vi "HOST_timecycling+4inputs.vi"() -> ()   [LabVIEW 2020]
uses:
  <vilib>/userDefined/Silver/nirio_resource_slv.ctl
  Controls/Clock Select.ctl
  <vilib>/FPGAPlugInAG/PXIe-7972R/niLvFpga_Open_PXIe-7972R.vi
  <vilib>/rvi/interface/common/dynamic/niFpgaDynamicAddResources.vi
  <vilib>/rvi/interface/common/niFpgaWaitOnOcc.vi
  <vilib>/Utility/error.llb/Error Cluster From Error Code.vi
  <vilib>/rvi/errors/niLvFpgaAdjustHostInterfaceError.vi
  <instrlib>/_niInstr/Streaming/v1/Host/Public/Start Finite Stream.vi
  <instrlib>/_niInstr/Streaming/v1/Host/Public/Wait for Stream.vi
  <instrlib>/_niInstr/Streaming/v1/Host/Public/Start Continuous Stream.vi
  <vilib>/FPGAPlugInAG/Dynamic/niLvFpga_Close_Dynamic.vi
  <vilib>/rvi/interface/nirviOpenFPGA/nirviOpenFPGA.xnode
  FPGA Bitfiles/rfsignal_FPGATarget_timecycling+4inp_VE6nLnBZ2oA.lvbitx
  <vilib>/rvi/interface/nirviMethod/nirviMethod.xnode
  <vilib>/rvi/interface/nirviReadWriteControl/nirviReadWriteControl.xnode
  <vilib>/rvi/interface/nirviCloseFPGA/nirviCloseFPGA.xnode
  <vilib>/rvi/errors/niLvFpgaMergeErrorWithErrorCode.vi
  <instrlib>/_niInstr/Streaming/v1/Host/niInstr Streaming v1 Host.lvlib
  <vilib>/rvi/interface/Simulation/niFpgaSimulationCallBeginRW.vi
  NiFpgaLv.dll
  <vilib>/FPGAPlugInAG/Dynamic/niLvFpga_ConfigureFifo_Dynamic.vi
  <vilib>/FPGAPlugInAG/Dynamic/niLvFpga_StartFifo_Dynamic.vi
  <vilib>/FPGAPlugInAG/Dynamic/niLvFpga_WriteFifo_Dynamic.vi
panel:
  in  "Feedback on/off":bool=TRUE
  in  "Scaling (Z)":fxp<+,5,-13>=9.918212890625e-05
  in  "Scaling (Y)":fxp<+,5,-13>=9.918212890625e-05
  in  "Scaling (X)":fxp<+,5,-13>=9.918212890625e-05
  in  "D (Z)":fxp<+/-,16,16>
  in  "I (Z)":fxp<+/-,16,16>
  in  "P (Z)":fxp<+/-,16,16>
  in  "D (Y)":fxp<+/-,16,16>
  in  "I (Y)":fxp<+/-,16,16>
  in  "P (Y)":fxp<+/-,16,16>
  in  "D (X)":fxp<+/-,16,16>
  in  "I (X)":fxp<+/-,16,16>
  in  "P (X)":fxp<+/-,16,16>
  in  "Gain X dec":bool
  in  "Gain X inc":bool
  in  "Gain X %/s":fxp<+/-,64,32>
  in  "Gain Y dec":bool
  in  "Gain Y inc":bool
  in  "Gain Y %/s":fxp<+/-,64,32>
  in  "X dec":bool
  in  "X inc":bool
  in  "X (CH1) Hz/s":fxp<+/-,64,32>
  in  "Y dec":bool
  in  "Y inc":bool
  in  "Y (CH0) Hz/s":fxp<+/-,64,32>
  in  "Input pass through\nmode":enum16{"Wire", "Accum", "Accum-edge"}(ring)
  in  "Ch 1 # of waves":i8=1
  in  "Ch 0 # of waves":i8=1
  in  "Wave Reader CH 1 (X)":fxp<+/-,64,32>[](array[numeric])=[27000000.0, 28000000.0, 28000000.0, 32000000.0, 21000000.0, 25000000.0, 30000000.0, 34000000.0] format="%_6p"
  in  "Gain CH 1 (multiplicative)":fxp<+,32,4>[](array[numeric])=[0.8999999985098839, 1.3999999985098839, 0.9999999925494194, 1.300000000745058, 1.0, 1.0, 1.0, 1.0]
  in  "Clean 2x edge cycles":i32=5
  in  "Time per beam in us":i32=100
  in  "stop":bool
  in  "Gain CH 0 (multiplicative)":fxp<+,32,4>[](array[numeric])=[0.8999999985098839, 0.6999999992549419, 1.199999999254942, 0.5, 1.0, 1.0, 1.0, 1.0]
  in  "Wave Reader CH 0 (Y)":fxp<+/-,64,32>[](array[numeric])=[27000000.0, 24000000.0, 28000000.0, 32000000.0, 21000000.0, 25000000.0, 30000000.0, 34000000.0] format="%_6p"
  out "AO":waveform(dbl)(graph)={"t0"=timestamp(0.0056 s since 1904-01-01), "dt"=1.220703125e-08, "Y"=array[65536 elements]}
  in  "Magnitude Initialization\nVpp":dbl[](array[numeric])=[1.0, 1.0] format="%0.2p"
  in  "Frequencies (Hz)":dbl[](array[numeric])=[10000.0, 10000.0] format="%5.0p"
  in  "Signal Type":T1(ring)
  in  "Sampling Info":cluster{"Fs":dbl, "#s":dbl}={"Fs"=163840000.0, "#s"=65536.0} {"Fs" format="%#_5p"}
  out "Error Out":errorcluster
  in  "Update Waveform":bool
  in  "AO Channel":T2(ring)
  in  "Clock Select":T3 items=["Internal Clock", "Internal Clock w/ Ref via CLK/REF IN", "Internal Clock w/ Ref via Sync Clock", "External Clock via CLK/REF IN"]
  in  "Rate of External Sample Clock (MHz)":u16=100 min=60 max=100 step=1
  in  "RIO Resource":T4="PXI1Slot5"
  # "Analog In"
  # "Waveform Initialization"
  # "Ch 1 Output Waveforms"
  # "Ch 0 Output Waveforms"
  # "DO NOT CHANGE"
  # "Ch0"
  # "Ch1"
  # "Don't change"
  # "Feedback parameters"
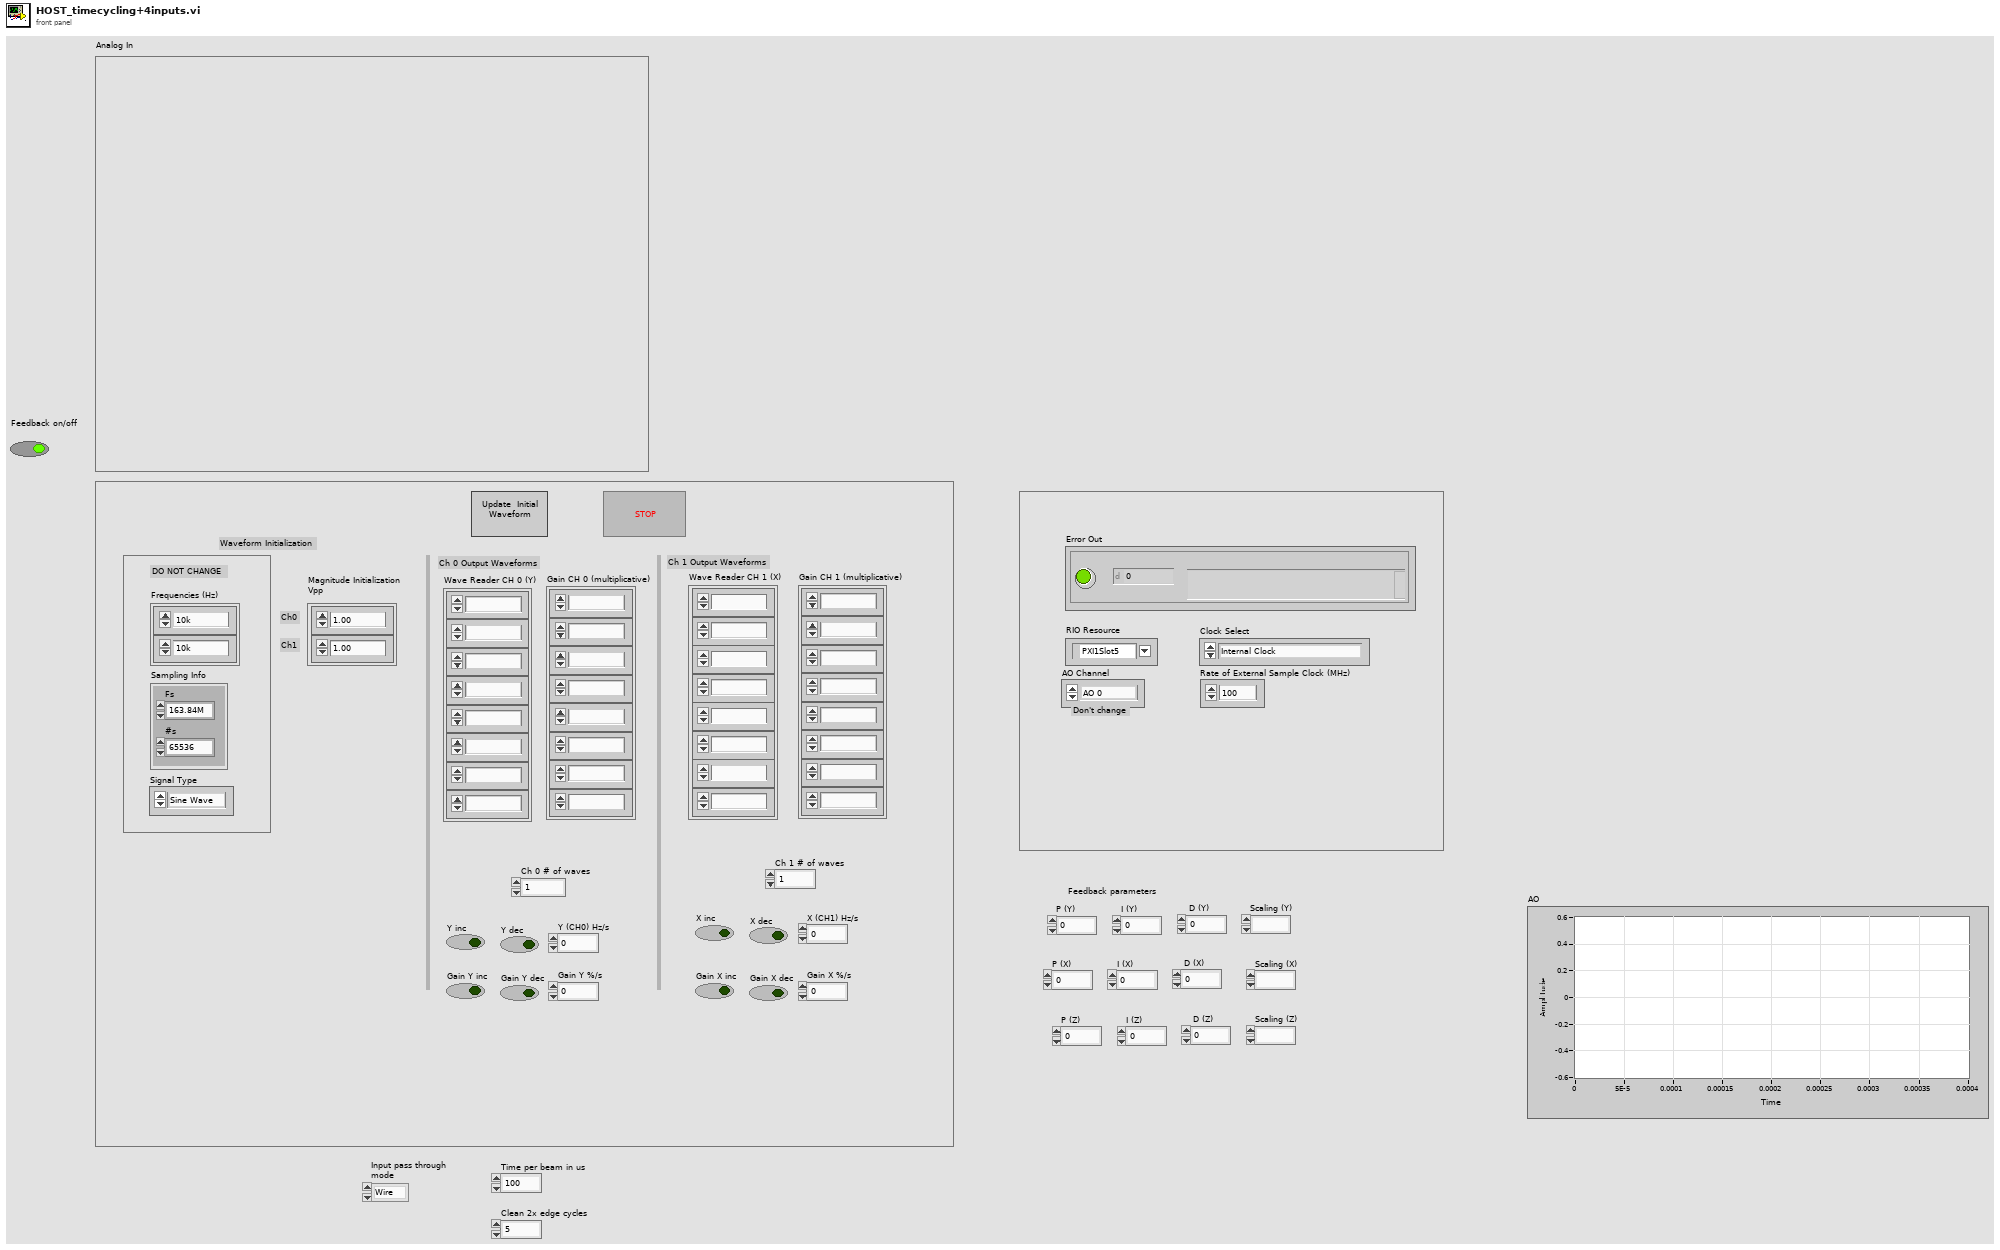
[diagram p1: front panel]
types:
  T1 = enum16{"Sine Wave", "Triangle Wave", "Square Wave", "Sawtooth Wave"}
  T2 = enum8{"AO 0", "AO 1", "AO 2", "AO 3", "AO 0, AO 1, AO 2, AO 3", "None"}
  T3 = typedef "Clock Select.ctl" = u16
  T4 = typedef "nirio_resource_slv.ctl" = tag
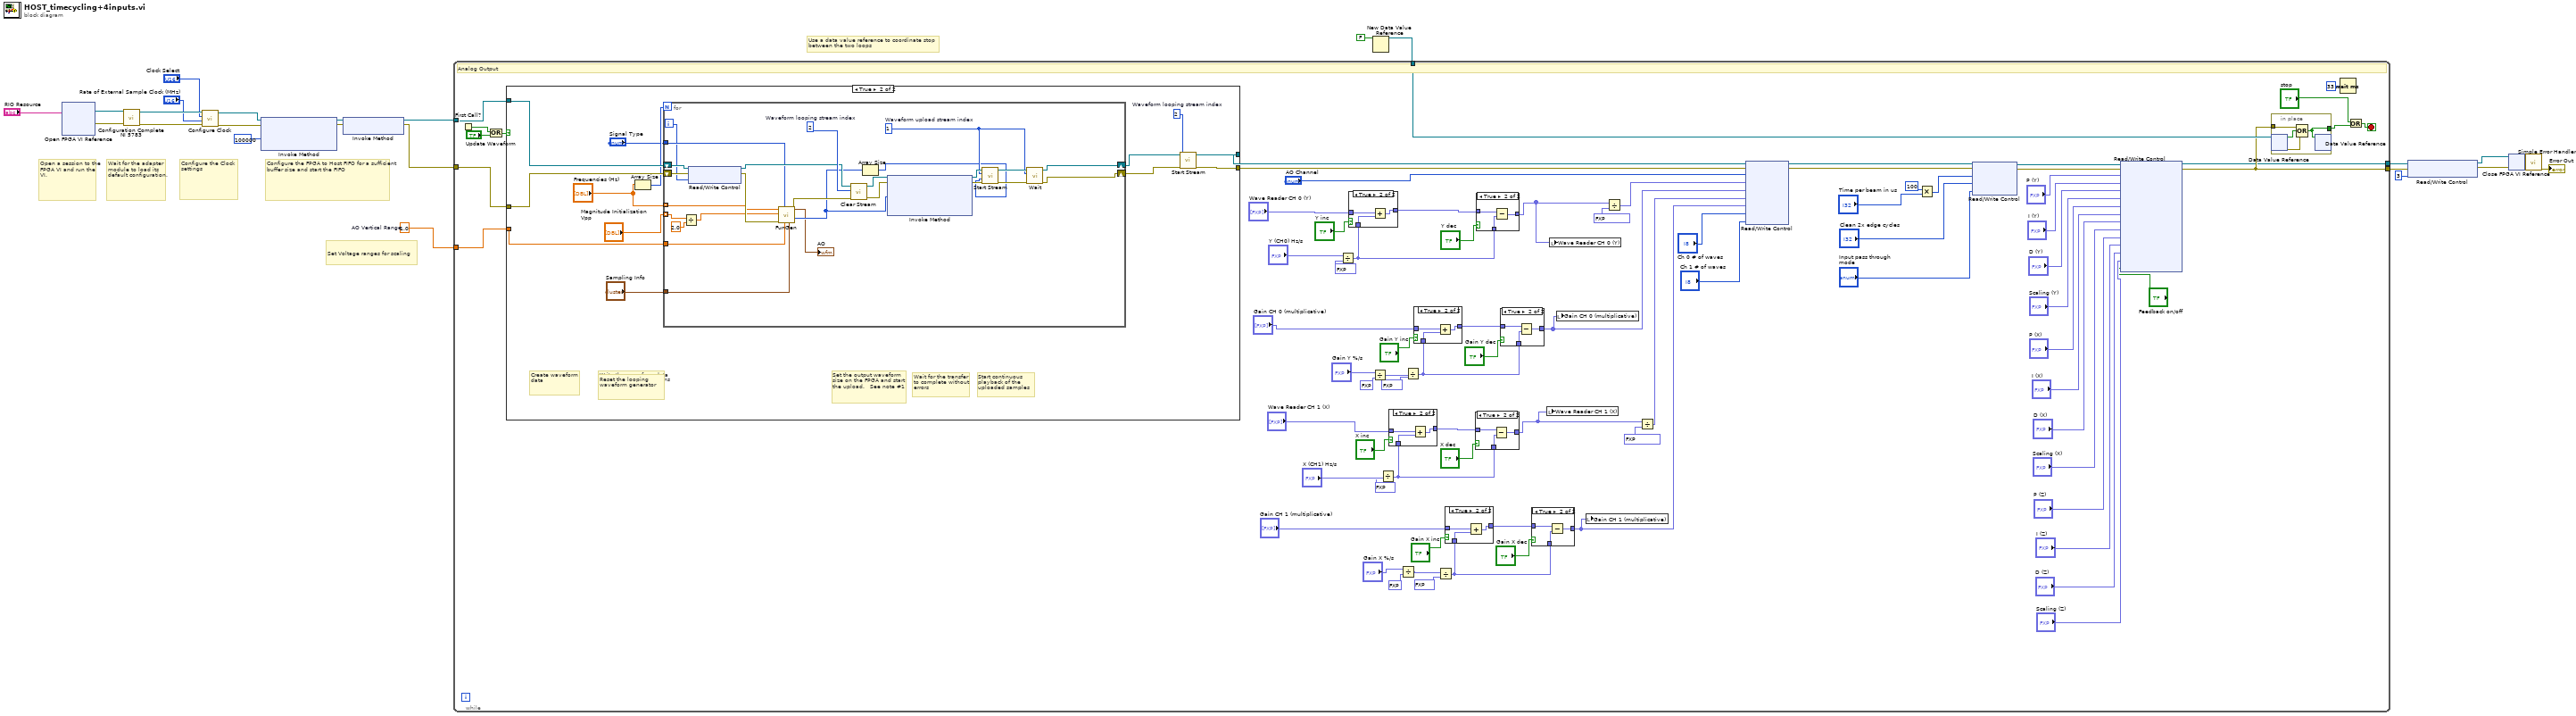
[diagram p0: block diagram]
diagram:
  w12 = 1.0  # AO Vertical Range
  # "Use a data value reference to coordinate stop between the two loops"
  # "Set Voltage ranges for scaling"
  # "Configure the Clock settings"
  # "Configure the FPGA to Host FIFO for a sufficient buffer size and start the FIFO"
  # "Wait for the adapter module to load its default configuration."
  # "Open a session to the FPGA VI and run the VI."
  n1 = xnode "Open FPGA VI Reference"("resource name"="RIO Resource") -> ("FPGA VI Reference Out"=w10:refnum<k20>, "error out"=w9:errorcluster)  [unwired: 1 in]
  n2 = call "Configuration Complete NI 5783.vi"("error in"=w9, "FPGA VI Reference In"=w10) -> ("error out"=w20:errorcluster, "FPGA VI Reference Out"=w21:refnum<k20>)  [unwired: 7 in, 1 out]
  n3 = call "Configure Clock.vi"("error in (no error)"=w20, "Rate of External Sample Clock (MHz)"="Rate of External Sample Clock (MHz)", "Clock Select"="Clock Select", "FPGA VI Reference In"=w21) -> ("error out"=w18:errorcluster, "FPGA VI Reference Out"=w19:refnum<k20>)  [unwired: 3 in, 3 out]
  n4 = xnode "Invoke Method"("FPGA VI Reference In"=w19, "error in"=w18, "Requested Depth"=u32 100000) -> ("FPGA VI Reference Out"=w24:refnum<k20>, "error out"=w23:errorcluster)  [unwired: 1 out]
  n5 = xnode "Invoke Method"("FPGA VI Reference In"=w24, "error in"=w23) -> ("FPGA VI Reference Out"=w3:refnum<k20>, "error out"=w2:errorcluster)
  n6 = New Data Value Reference(data value=FALSE ("Stopped")) -> (data value reference=w1:refnum<data-value>)  [unwired: 1 in, 1 out]
  n7 = while {
    tunnel: w2 -> [w98]
    tunnel: [w43] -> w8
    tunnel: w3 -> [w104]
    tunnel: [w42] -> w7
    tunnel: w1 -> [w99]
    tunnel: w12 -> [w97]
    stop <- w93 stop-if-true
    # "Analog Output"
    n8 = First Call?() -> (First Call?: T/F=w100:bool)
    n9 = Or(x=w100, y="Update Waveform") -> (x .or. y?=w101:bool)
    n10 = case shown="True" w101 {
      tunnel: [w142 w155] -> w96
      tunnel: [w141 w154] -> w95
      tunnel: w104 -> [w142 w152]
      tunnel: w98 -> [w141 w151]
      tunnel: w97 -> [_ w153]
      frame False {
      }
      frame True {
        w150 = 2  # Waveform looping stream index
        # "Loop over the waveforms to combine"
        # "Reset the looping waveform generator"
        # "Start continuous playback of the uploaded samples"
        # "Wait for the transfer to complete without errors"
        # "Set the output waveform size on the FPGA and start the upload.   See note #1"
        # "Write the waveform data to the FPGA for generation"
        # "Create waveform data"
        n11 = Array Size(array="Frequencies (Hz)") -> (size(s)=w145:i32)
        n12 = for {
          N: w145 -> [_]
          tunnel: w153 -> [w171]
          shift-right: [w165] -> w149
          shift-left: w152 -> [w170]
          shift-right: [w164] -> w148
          shift-left: w151 -> [w168]
          tunnel: "Frequencies (Hz)" -> [w163] mode=indexing
          tunnel: "Magnitude Initialization\nVpp" -> [w159] mode=indexing
          tunnel: "Sampling Info" -> [w162]
          tunnel: "Signal Type" -> [w161]
          i -> [w160]
          w172 = 2  # Waveform looping stream index
          w177 = 1  # Waveform upload stream index
          n13 = Divide(x=w159, y=2.0) -> (x/y=w158:dbl)
          n14 = xnode "Read/Write Control"("FPGA VI Reference In"=w170, "error in"=w168, "Upload selector"=w160) -> ("FPGA VI Reference Out"=w169:refnum<k20>, "error out"=w167:errorcluster)
          n15 = call "FunGen.vi"("sampling info"=w162, "range (Vpp)"=w171, "signal type"=w161, "error in (no error)"=w167, "amplitude"=w158, "frequency"=w163) -> ("error out"=w173:errorcluster, "Waveform Data"=w166:i16[], "Output Waveform (V)"=→"AO":waveform(dbl))  [unwired: 2 in, 1 out]
          n16 = call <instrlib>:"Clear Stream.vi"("error in (no error)"=w173, "stream index"=w172, "refnum in"=w169) -> ("error out"=w175:errorcluster, "refnum out"=w176:refnum<k20>)  [unwired: 7 in]
          n17 = Array Size(array=w166) -> (size(s)=w174:i32)
          n18 = xnode "Invoke Method"("FPGA VI Reference In"=w176, "error in"=w175, "Data"=w166) -> ("FPGA VI Reference Out"=w181:refnum<k20>, "error out"=w180:errorcluster)  [unwired: 1 in, 1 out]
          n19 = call-poly <instrlib>:"Start Stream.vi"("error in (no error)"=w180, "num samples"=w174, "stream index"=w177, "refnum in"=w181) -> ("error out"=w178:errorcluster, "refnum out"=w179:refnum<k20>)  [unwired: 6 in]
          n20 = call-poly <instrlib>:"Wait.vi"("error in (no error)"=w178, "stream index"=w177, "refnum in"=w179) -> ("error out"=w164:errorcluster, "refnum out"=w165:refnum<k20>)  [unwired: 5 in, 2 out]
        }
        n21 = call-poly <instrlib>:"Start Stream.vi"("error in (no error)"=w148, "stream index"=w150, "refnum in"=w149) -> ("error out"=w154:errorcluster, "refnum out"=w155:refnum<k20>)  [unwired: 7 in]
      }
    }
    n22 = Divide(x="Y (CH0) Hz/s", y=fxp<+,20,5> 30.303009033203125) -> (x/y=w72:fxp<+/-,64,32>)
    n23 = case shown="True" "Y inc" {
      tunnel: "Wave Reader CH 0 (Y)" -> [w133 w136]
      tunnel: [w133 w135] -> w76
      tunnel: w72 -> [_ w134]
      frame False {
      }
      frame True {
        n24 = Add(x=w136, y=w134) -> (x+y=w135:fxp<+/-,64,32>[])
      }
    }
    n25 = Divide(x="Gain Y %/s", y=fxp<+,5,7> 100.0) -> (x/y=w47:fxp<+/-,64,32>)
    n26 = Divide(x="X (CH1) Hz/s", y=fxp<+,20,5> 30.303009033203125) -> (x/y=w66:fxp<+/-,64,32>)
    n27 = case shown="True" "X inc" {
      tunnel: "Wave Reader CH 1 (X)" -> [w125 w128]
      tunnel: [w125 w127] -> w70
      tunnel: w66 -> [_ w126]
      frame False {
      }
      frame True {
        n28 = Add(x=w128, y=w126) -> (x+y=w127:fxp<+/-,64,32>[])
      }
    }
    n29 = Divide(x="Gain X %/s", y=fxp<+,5,7> 100.0) -> (x/y=w51:fxp<+/-,64,32>)
    n30 = Divide(x=w47, y=fxp<+,20,5> 30.303009033203125) -> (x/y=w60:fxp<+/-,64,32>)
    n31 = case shown="True" "Gain Y inc" {
      tunnel: "Gain CH 0 (multiplicative)" -> [w117 w120]
      tunnel: [w117 w119] -> w63
      tunnel: w60 -> [_ w118]
      frame False {
      }
      frame True {
        n32 = Add(x=w120, y=w118) -> (x+y=w119:fxp<+,32,4>[])
      }
    }
    n33 = Divide(x=w51, y=fxp<+,20,5> 30.303009033203125) -> (x/y=w54:fxp<+/-,64,32>)
    n34 = case shown="True" "Gain X inc" {
      tunnel: "Gain CH 1 (multiplicative)" -> [w109 w112]
      tunnel: [w109 w111] -> w57
      tunnel: w54 -> [_ w110]
      frame False {
      }
      frame True {
        n35 = Add(x=w112, y=w110) -> (x+y=w111:fxp<+,32,4>[])
      }
    }
    n36 = case shown="True" "X dec" {
      tunnel: w70 -> [w121 w124]
      tunnel: w66 -> [_ w123]
      tunnel: [w121 w122] -> w26
      frame False {
      }
      frame True {
        n37 = Subtract(x=w124, y=w123) -> (x-y=w122:fxp<+/-,64,32>[])
      }
    }
    n38 = case shown="True" "Y dec" {
      tunnel: w76 -> [w129 w132]
      tunnel: w72 -> [_ w131]
      tunnel: [w129 w130] -> w28
      frame False {
      }
      frame True {
        n39 = Subtract(x=w132, y=w131) -> (x-y=w130:fxp<+/-,64,32>[])
      }
    }
    n40 = case shown="True" "Gain Y dec" {
      tunnel: w63 -> [w113 w116]
      tunnel: w60 -> [_ w115]
      tunnel: [w113 w114] -> w27
      frame False {
      }
      frame True {
        n41 = Subtract(x=w116, y=w115) -> (x-y=w114:fxp<+,32,4>[])
      }
    }
    n42 = case shown="True" "Gain X dec" {
      tunnel: w57 -> [w105 w108]
      tunnel: w54 -> [_ w107]
      tunnel: [w105 w106] -> w25
      frame False {
      }
      frame True {
        n43 = Subtract(x=w108, y=w107) -> (x-y=w106:fxp<+,32,4>[])
      }
    }
    n44 = local write "Wave Reader CH 1 (X)"(w26) -> ()
    n45 = local write "Wave Reader CH 0 (Y)"(w28) -> ()
    n46 = local write "Gain CH 0 (multiplicative)"(w27) -> ()
    n47 = local write "Gain CH 1 (multiplicative)"(w25) -> ()
    n48 = Divide(x=w28, y=fxp<+,32,16> 6103.515625) -> (x/y=w84:fxp<+,32,16>[])
    n49 = Divide(x=w26, y=fxp<+,32,16> 6103.515625) -> (x/y=w82:fxp<+,32,16>[])
    n50 = xnode "Read/Write Control"("FPGA VI Reference In"=w96, "error in"=w95, "AO Channel"="AO Channel", "Wave 1"=w84, "Amp 1"=w27, "Wave 2"=w82, "Amp 2"=w25, "Ch 0 size"="Ch 0 # of waves", "Ch 1 size"="Ch 1 # of waves") -> ("FPGA VI Reference Out"=w89:refnum<k20>, "error out"=w88:errorcluster)
    n51 = Multiply(x=100, y="Time per beam in us") -> (x*y=w85:i32)
    n52 = xnode "Read/Write Control"("FPGA VI Reference In"=w89, "error in"=w88, "Timeshare"=w85, "Edge size"="Clean 2x edge cycles", "Pass selector"="Input pass through\nmode") -> ("FPGA VI Reference Out"=w45:refnum<k20>, "error out"=w44:errorcluster)
    n53 = xnode "Read/Write Control"("FPGA VI Reference In"=w45, "error in"=w44, "P gain 1"="P (Y)", "I gain 1"="I (Y)", "D gain 1"="D (Y)", "Feedback scaling"="Scaling (Y)", "P gain 2"="P (X)", "D gain 2"="I (X)", "I gain 2"="D (X)", "Feedback scaling 2"="Scaling (X)", "P gain 3"="P (Z)", "D gain 3"="I (Z)", "I gain 3"="D (Z)", "Feedback scaling 3"="Scaling (Z)", "Feedback on/off"="Feedback on/off") -> ("FPGA VI Reference Out"=w42:refnum<k20>, "error out"=w43:errorcluster)
    n54 = in-place {
      in-place-border: [w138] -> w92
      in-place-border: w43 -> [w140]
      n55 = in-place-dvr #1(w99) -> (w139:bool, w137:errorcluster)
      n56 = Compound Arithmetic op=OR(w140, w139, w137) -> (w138:bool)
      n57 = in-place-dvr #1(w138) -> ()  [unwired: 2 out]
    }
    n58 = Wait (ms)(milliseconds to wait=u32 33) -> ()  [unwired: 1 out]
    n59 = Or(x="stop", y=w92) -> (x .or. y?=w93:bool)
  }
  n60 = xnode "Read/Write Control"("FPGA VI Reference In"=w7, "error in"=w8, "stream.request state 2"=3) -> ("FPGA VI Reference Out"=w4:refnum<k20>, "error out"=w6:errorcluster)
  n61 = xnode "Close FPGA VI Reference"("FPGA VI Reference In"=w4, "error in"=w6) -> ("error out"=w15:errorcluster)
  n62 = call <vilib>:"Simple Error Handler.vi"("error in (no error)"=w15) -> ("error out"=→"Error Out":errorcluster)  [unwired: 4 in, 4 out]
